vi "Write Analog_Input.vi"(10 "Analog_Input.lvclass":refnum<class "Analog_Input.lvclass">, 11 "Experiment in":refnum<class "Experiment.lvclass">) -> (3 "Experiment out":refnum<class "Experiment.lvclass">)   [LabVIEW 2013, in "Experiment.lvclass"]
uses:
  Experiment.lvclass
  Analog_Input/Analog_Input.lvclass
  Experiment.lvclass/Experiment.ctl
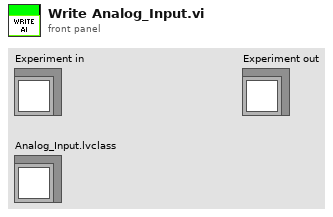
[diagram p1: front panel]
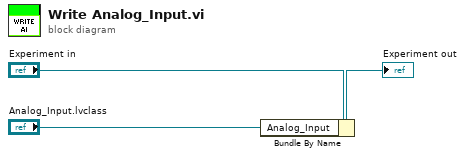
[diagram p0: block diagram]
diagram:
  n1 = Bundle By Name(cluster="Experiment in", "Analog_Input"="Analog_Input.lvclass") -> (→"Experiment out":refnum<class "Experiment.lvclass">)
